vi "how_many_seats.vi"(1 "selected seats before":i32[](array[numeric])) -> (0 "How many seats do \nyou want to choose?\n(O)":i32)   [LabVIEW 2014]
panel:
  in  "How many seats do \nyou want to choose?":i32
  in  "OK Button":bool
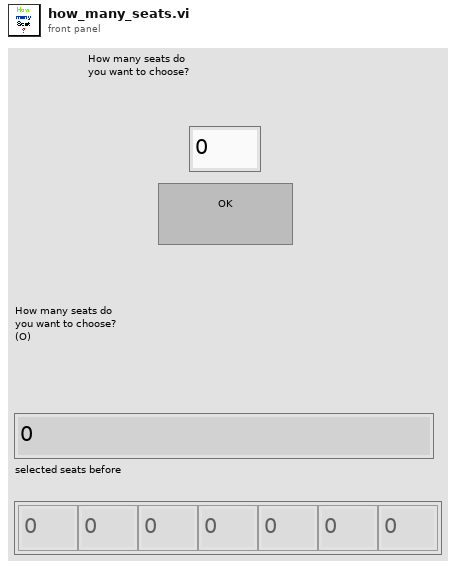
[diagram p1: front panel]
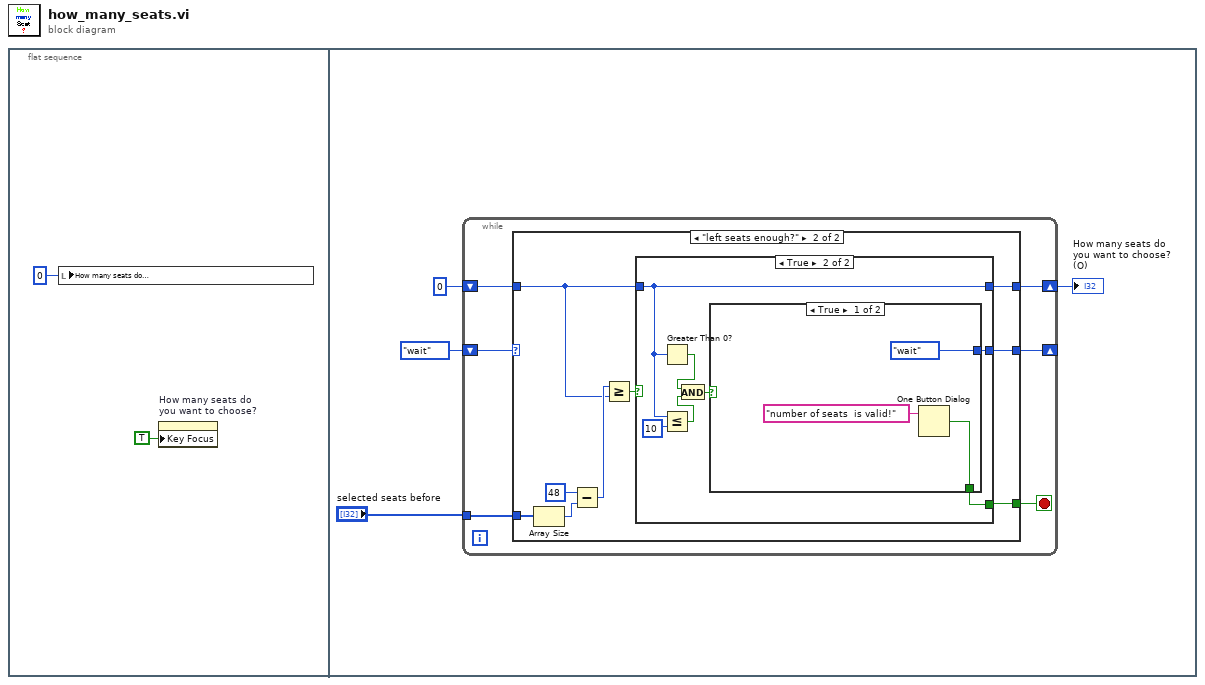
[diagram p0: block diagram]
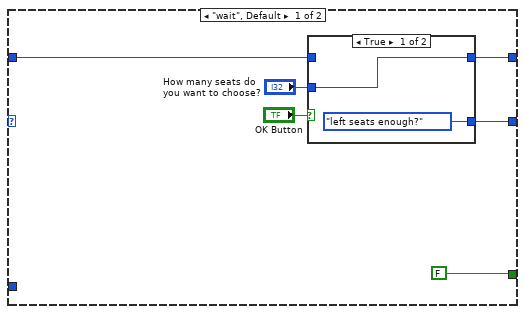
[diagram p2: hidden frame]
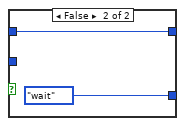
[diagram p3: hidden frame]
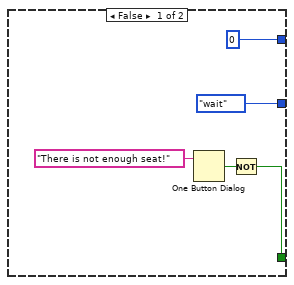
[diagram p4: hidden frame]
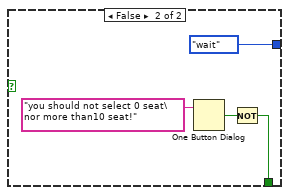
[diagram p5: hidden frame]
diagram:
  n1 = flat-sequence {
    frame #0 {
      n2 = local write "How many seats do \nyou want to choose?"(0 ("How many seats do \nyou want to choose?")) -> ()
      n3 = property on="How many seats do \nyou want to choose?" class="DigNum (strict)"("Key Focus"=TRUE) -> ()  [unwired: 2 in, 2 out]
    }
    frame #1 {
      n4 = while {
        tunnel: "selected seats before" -> [w11]
        shift-right: [w10] -> _
        shift-left: enum16{"wait", "left seats enough?"}."wait" -> [w12]
        shift-right: [w8] -> w4
        shift-left: 0 ("How many seats do you want to choose?") -> [w9]
        stop <- w7 stop-if-true
        n5 = case shown="\"left seats enough?\"" w12 {
          tunnel: w11 -> [_ w31]
          tunnel: [w17 w25] -> w10
          tunnel: w9 -> [w14 w23]
          tunnel: [w15 w24] -> w8
          tunnel: [FALSE w26] -> w7
          frame "wait", Default {
            n6 = case shown="True" "OK Button" {
              tunnel: [enum16{"wait", "left seats enough?"}."left seats enough?" enum16{"wait", "left seats enough?"}."wait"] -> w17
              tunnel: "How many seats do \nyou want to choose?" -> [w19 _]
              tunnel: [w19 w21] -> w15
              tunnel: w14 -> [_ w21]
              frame True {
              }
              frame False {
              }
            }
          }
          frame "left seats enough?" {
            n7 = Array Size(array=w31) -> (size(s)=w29:i32)
            n8 = Subtract(x=48, y=w29) -> (x-y=w27:i32)
            n9 = Greater Or Equal?(x=w27, y=w23) -> (x >= y?=w28:bool)
            n10 = case shown="True" w28 {
              tunnel: [w32 w42] -> w26
              tunnel: [enum16{"wait", "left seats enough?"}."wait" w43] -> w25
              tunnel: [0 w41] -> w24
              tunnel: w23 -> [_ w41]
              frame False {
                n11 = One Button Dialog(message="There is not enough seat!") -> (true=w33:bool)  [unwired: 1 in]
                n12 = Not(x=w33) -> (.not. x?=w32:bool)
              }
              frame True {
                n13 = Greater Than 0?(x=w41) -> (x > 0?=w38:bool)
                n14 = Less Or Equal?(x=w41, y=10) -> (x <= y?=w39:bool)
                n15 = And(x=w38, y=w39) -> (x .and. y?=w37:bool)
                n16 = case shown="True" w37 {
                  tunnel: [enum16{"wait", "left seats enough?"}."wait" enum16{"wait", "left seats enough?"}."wait"] -> w43
                  tunnel: [w44 w47] -> w42
                  frame True {
                    n17 = One Button Dialog(message="number of seats  is valid!") -> (true=w44:bool)  [unwired: 1 in]
                  }
                  frame False {
                    n18 = One Button Dialog(message="you should not select 0 seat\nor more than10 seat!") -> (true=w48:bool)  [unwired: 1 in]
                    n19 = Not(x=w48) -> (.not. x?=w47:bool)
                  }
                }
              }
            }
          }
        }
      }
      "How many seats do \nyou want to choose?\n(O)" <- w4
    }
  }
